vi "MM6.Initialize.vi"(0 "i ref in":refnum<vi>, 3 "ms timeout (10000)":i32=10000, 5 "error in (no error)":errorcluster) -> (14 "i ref out":refnum<vi>, 17 "timed out":bool, 19 "error out":errorcluster)   [LabVIEW 2014, in "MM6.lvlib"]
doc: "Initializes a measurement by loading and initializing the required objects."
uses:
  MM6.lvlib
  CS_Core/CSSystem/CoreDefs/CoreDefs.error_type.ctl
  CS_Core/CSSystem/CoreLib/CoreLib.lvlib
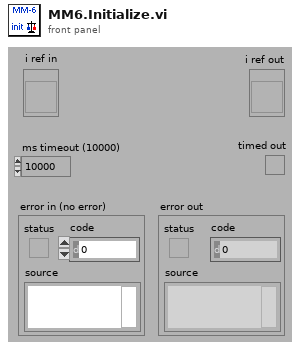
[diagram p1: front panel]
types:
  T1 = typedef "CoreDefs.error_type.ctl" = enum16{"no error", "can't load process", "can't unload process", "process does not exist", "can't install process", "can't remove process", "unknown function", "time out", "can't execute function", "duplicate queue name", "super not found", "caller queue invalid", "can't ping process", "unknown error", "VISA Error", "VISA timeout", "GPIB timeout", "GPIB error", "communication error", "data type mismatch", "can't read data from OPC server", "can't write data to OPC server", "OET error", "function not implemented", "process already exists", "invalid Shared Variable name", "error writing Shared Variable", "error reading Shared Variable", "invalid client name", "corrupt database", "unknown class", "call not authorized", "parameter out of range", "OET timeout: can't get data to modify", "invalid queue name", "requested operation incompatible with current state", "event undefined", "event disabled", "state undefined", "caller is not a friend", "EventBuilder: bad eventID", "EventBuilder: no DAQ devices", "a thread must not stop itself", "UNUSED ELEMENT4", "DiscArchiver: eventData incomplete", "DiscArchiver: eventData does not belong to run", "DiscArchiver: can't open file", "DiscArchiver: can't write to file", "DiscArchiver: available disc space low", "can't acquire semaphore", "error reading data from database", "notifier object is not existing", "can't register process", "can't unregister process", "illegal event type", "object disabled", "object already exists", "can't change state", "Instrument not found", "no connection to remote node", "invalid reference", "N/A", "UNUSED ELEMENT 1", "element not found", "illegal TCP/IP connection detected", "object does not exist", "invalid access ID", "unknown CS system", "invalid privilige", "unsupported data type", "unsupported server type", "IO server already exists", "Shared Variable already exists"}
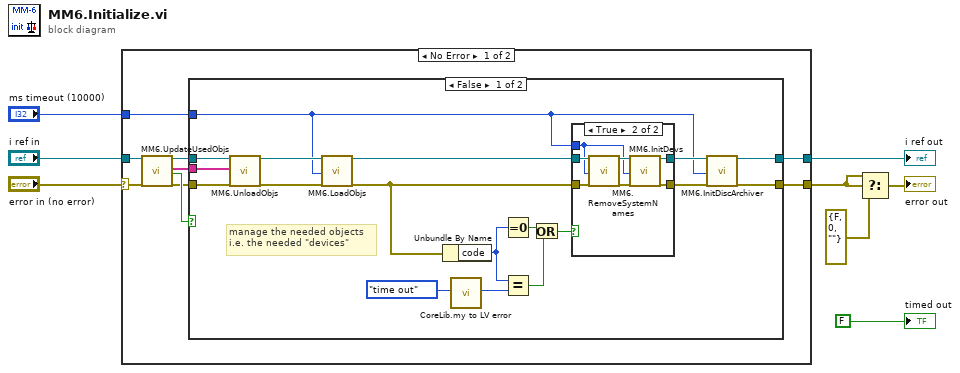
[diagram p0: block diagram]
diagram:
  n1 = case shown="No Error" "error in (no error)" {
    selector: "error in (no error)" -> [w11 w48]
    tunnel: "i ref in" -> [w17 w47]
    tunnel: [w13 w47] -> w2
    tunnel: [w12 w48] -> w6
    tunnel: "ms timeout (10000)" -> [w9 _]
    frame No Error {
      n2 = call "MM6.UpdateUsedObjs.vi"("i ref in"=w17, "error in (no error)"=w11) -> ("i ref out"=w15:refnum<vi>, "UnusedObjs"=w10:string[], "timed out"=w16:bool, "error out"=w14:errorcluster)  [unwired: 14 in]
      n3 = case shown="False" w16 {
        tunnel: w15 -> [w28 w46]
        tunnel: w14 -> [w27 w45]
        tunnel: [w20 w46] -> w13
        tunnel: [w19 w45] -> w12
        tunnel: w10 -> [w23 _]
        tunnel: w9 -> [w18 _]
        frame False {
          # "manage the needed objects\ni.e. the needed \"devices\""
          n4 = call "MM6.UnloadObjs.vi"("i ref in"=w28, "ObjsToUnload"=w23, "error in (no error)"=w27) -> ("i ref out"=w35:refnum<vi>, "error out"=w34:errorcluster)  [unwired: 15 in]
          n5 = call "MM6.LoadObjs.vi"("i ref in"=w35, "ms timeout (10000)"=w18, "error in (no error)"=w34) -> ("i ref out"=w26:refnum<vi>, "error out"=w25:errorcluster)  [unwired: 14 in, 1 out]
          n6 = Unbundle By Name(w25) -> ("code"=w30:i32)
          n7 = call "CoreLib.my to LV error.vi"("ErrorTypes"=CoreDefs.error_type."time out") -> ("LV error code"=w32:i32)  [unwired: 17 in, 1 out]
          n8 = Equal To 0?(x=w30) -> (x = 0?=w31:bool)
          n9 = Equal?(x=w30, y=w32) -> (x = y?=w29:bool)
          n10 = Or(x=w31, y=w29) -> (x .or. y?=w24:bool)
          n11 = case shown="True" w24 {
            tunnel: w26 -> [w37 w42]
            tunnel: w25 -> [w36 w39]
            tunnel: [w37 w44] -> w22
            tunnel: [w36 w43] -> w21
            tunnel: w18 -> [_ w38]
            frame False {
            }
            frame True {
              n12 = call "MM6.RemoveSystemNames.vi"("i ref in"=w42, "ms timeout (10000)"=w38, "error in (no error)"=w39) -> ("i ref out"=w41:refnum<vi>, "error out"=w40:errorcluster)  [unwired: 14 in, 1 out]
              n13 = call "MM6.InitDevs.vi"("i ref in"=w41, "ms timeout (10000)"=w38, "error in (no error)"=w40) -> ("i ref out"=w44:refnum<vi>, "error out"=w43:errorcluster)  [unwired: 14 in, 1 out]
            }
          }
          n14 = call "MM6.InitDiscArchiver.vi"("i ref in"=w22, "ms timeout (10000)"=w18, "error in (no error)"=w21) -> ("i ref out"=w20:refnum<vi>, "error out"=w19:errorcluster)  [unwired: 14 in, 1 out]
        }
        frame True {
        }
      }
    }
    frame Error {
    }
  }
  "i ref out" <- w2
  n15 = Select(t=w6, s=w6, f=errorcluster {"status"=FALSE, "code"=0, "source"=""} ("error out")) -> (s? t:f=→"error out":errorcluster)
  "timed out" <- FALSE ("timed out")
